vi "试剂余量后台任务.vi"   [LabVIEW 2016, in "斯坦道总氮.lvlib"]
uses:
  <vilib>/ptbypt/NI_PtbyPt.lvlib
types:
  T1 = cluster{"V1":sgl, "V2":sgl, "V3":sgl, "V4":sgl, "V5":sgl, "V6":sgl, "V7":sgl, "V8":sgl, "V9":sgl, "V10":sgl, "V11":sgl, "V12":sgl, "V9-1":sgl, "V9-2":sgl}
  T2 = cluster{"时间标识":timestamp, "设备":string, "日志信息":string, "备注":string}
  T3 = cluster{"系统时间":timestamp, "工作状态":u16, "测量模式":enum16{"待机", "连续模式", "周期模式", "定点模式", "受控模式", "手动模式"}, "告警代码":u16, "故障代码":u16, "日志代码":u16, "软件版本":u16, "F0":sgl, "F1":sgl, "F2":sgl, "F3":sgl, "T":sgl, "H":sgl, "id":u16, "flowid":u16, "量程":u16, "总磷控温温度1":sgl, "营养盐控温温度2":sgl, "ADC":sgl}
  T4 = cluster{"V1":bool, "V2":bool, "V3":bool, "V4":bool, "V5":bool, "V6":bool, "V7":bool, "V8":bool, "V9":bool, "V10":bool, "V11":bool, "V12":bool, "V9-1":bool, "V9-2":bool}
  T5 = cluster{"参数":string, "报警内容":string, "报警分析":string}
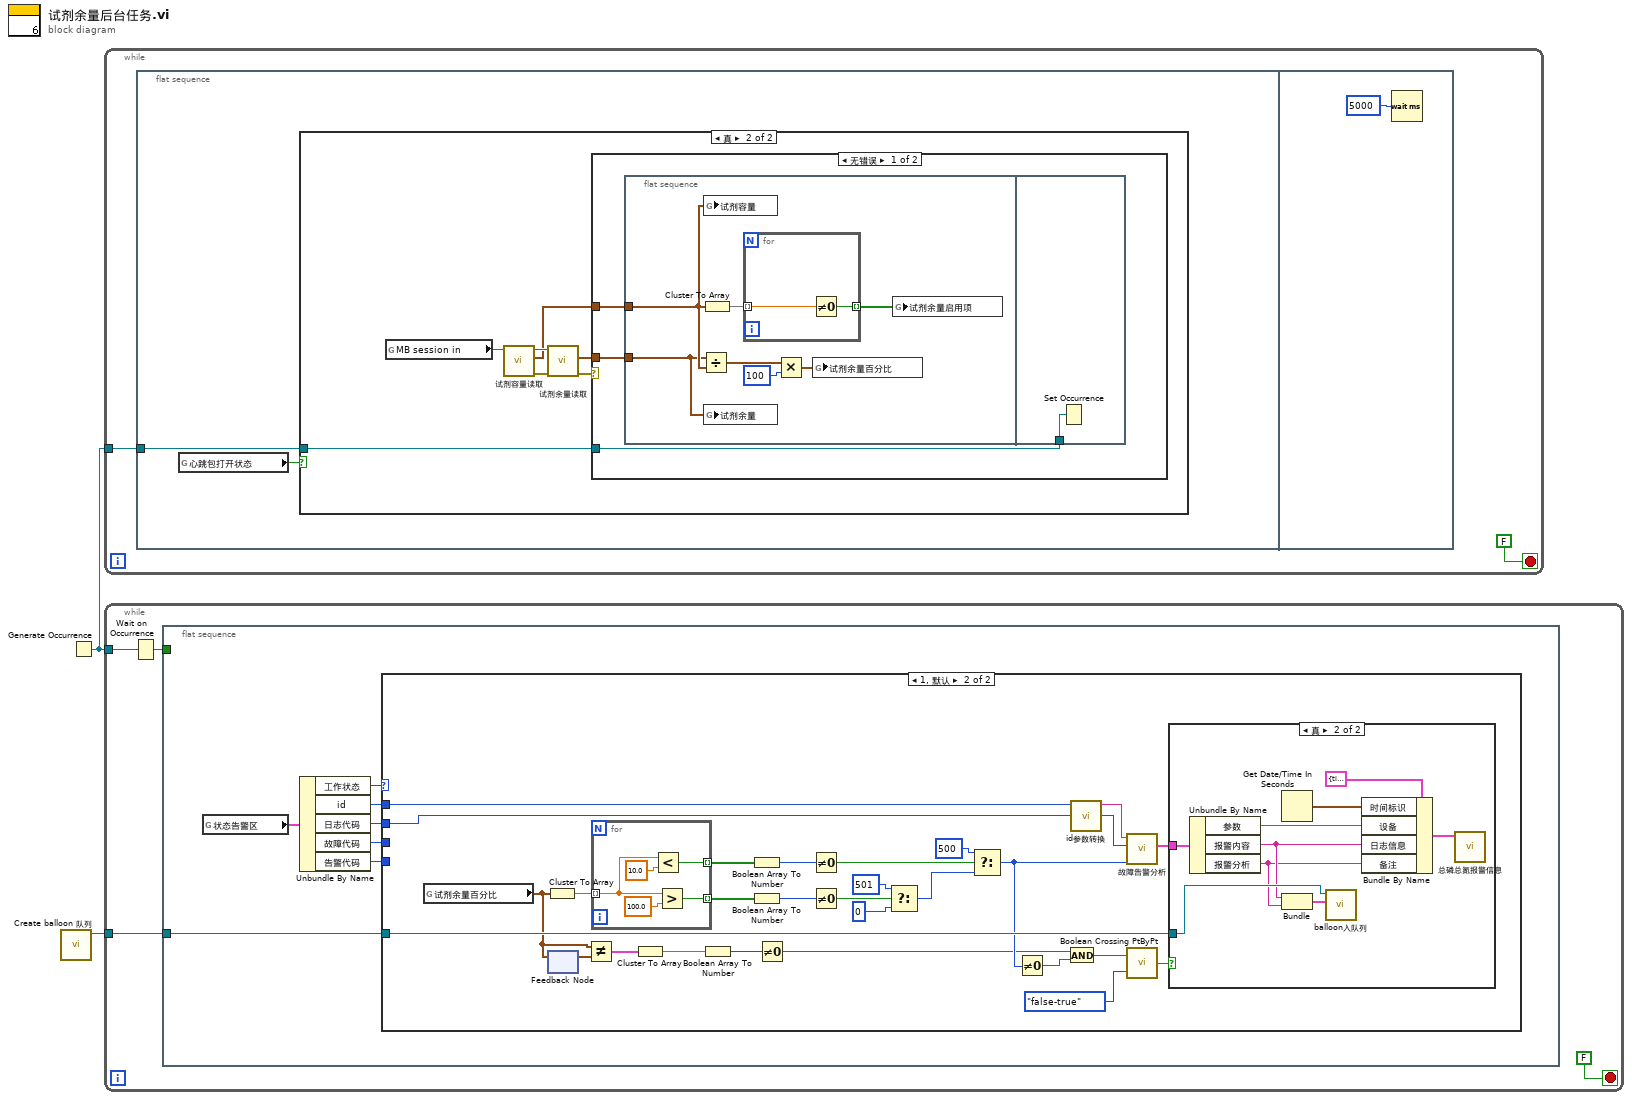
[diagram p0: block diagram]
diagram:
  n1 = call "Create balloon 队列.vi"() -> ("队列输出"=w2:refnum<queue>)  [unwired: 11 in]
  n2 = Generate Occurrence() -> (w1:refnum<k4>)
  n3 = while {
    tunnel: w1 -> [w3]
    stop <- FALSE stop-if-true
    n4 = flat-sequence {
      tunnel: w3 -> [w6]
      frame #0 {
        n5 = global read "VAR总磷总氮全局变量.vi" "心跳包打开状态"() -> (w5:bool)
        n6 = case shown="真" w5 {
          tunnel: w6 -> [_ w7]
          frame False {
          }
          frame True {
            n7 = global read "VAR总磷总氮全局变量.vi" "MB session in"() -> (w11:refnum<class "MB_Master.lvclass">)
            n8 = call "试剂容量读取.vi"("MB session in"=w11) -> ("error out"=w13:errorcluster, "试剂容量"=w10:T1, "MB session out"=w12:refnum<class "MB_Master.lvclass">)  [unwired: 8 in]
            n9 = call "试剂余量读取.vi"("Error in"=w13, "MB session in"=w12) -> ("error out"=w8:errorcluster, "试剂余量"=w9:T1)  [unwired: 7 in, 1 out]
            n10 = case shown="无错误" w8 {
              tunnel: w10 -> [w16 _]
              tunnel: w9 -> [w15 _]
              tunnel: w7 -> [w14 _]
              frame No Error {
                n11 = flat-sequence {
                  tunnel: w16 -> [w21]
                  tunnel: w15 -> [w20]
                  tunnel: w14 -> [w26]
                  frame #0 {
                    n12 = Divide(x=w20, y=w21) -> (x/y=w23:T1)
                    n13 = Cluster To Array(cluster=w21) -> (array=w18:sgl[])
                    n14 = global write "VAR总磷总氮全局变量.vi" "试剂容量"(w21) -> ()
                    n15 = global write "VAR总磷总氮全局变量.vi" "试剂余量"(w20) -> ()
                    n16 = for {
                      tunnel: w18 -> [w25] mode=indexing
                      tunnel: [w24] -> w17 mode=indexing
                      n17 = Not Equal To 0?(x=w25) -> (x != 0?=w24:bool)
                    }
                    n18 = Multiply(x=w23, y=100) -> (x*y=w19:T1)
                    n19 = global write "VAR总磷总氮全局变量.vi" "试剂余量百分比"(w19) -> ()
                    n20 = global write "VAR总磷总氮全局变量.vi" "试剂余量启用项"(w17) -> ()
                  }
                  frame #1 {
                    n21 = Set Occurrence(w26) -> ()
                  }
                }
              }
              frame Error {
              }
            }
          }
        }
      }
      frame #1 {
        n22 = Wait (ms)(milliseconds to wait=u32 5000 ("等待时间（毫秒）")) -> ()  [unwired: 1 out]
      }
    }
  }
  n23 = while {
    tunnel: w2 -> [w30]
    tunnel: w1 -> [w29]
    stop <- FALSE stop-if-true
    n24 = Wait on Occurrence(2:w29) -> (0:w28:bool)  [unwired: 2 in]
    n25 = flat-sequence {
      tunnel: w30 -> [w36]
      tunnel: w28 -> [_]
      frame #0 {
        n26 = global read "VAR总磷总氮全局变量.vi" "状态告警区"() -> (w32:T3)
        n27 = Unbundle By Name(w32) -> ("工作状态"=w33:u16, "id"=w38:u16, "日志代码"=w37:u16, "故障代码"=w35:u16, "告警代码"=w34:u16)
        n28 = case shown="1, 默认" w33 {
          tunnel: w38 -> [_ w65]
          tunnel: w37 -> [_ w64]
          tunnel: w36 -> [_ w61]
          tunnel: w35 -> [_ _]
          tunnel: w34 -> [_ _]
          frame 0 {
          }
          frame 1, Default {
            n29 = global read "VAR总磷总氮全局变量.vi" "试剂余量百分比"() -> (w46:T1)
            n30 = Cluster To Array(cluster=w46) -> (array=w56:sgl[])
            n31 = feedback-in #1(w46) -> ()
            n32 = feedback #1() -> (w47:T1)  [unwired: 1 in]
            n33 = Not Equal?(x=w46, y=w47) -> (x != y?=w45:T4)
            n34 = for {
              tunnel: w56 -> [w68] mode=indexing
              tunnel: [w69] -> w58 mode=indexing
              tunnel: [w66] -> w57 mode=indexing
              n35 = Less?(x=w68, y=sgl 10.0) -> (x < y?=w69:bool)
              n36 = Greater?(x=w68, y=sgl 100.0) -> (0:w66:bool)
            }
            n37 = Cluster To Array(cluster=w45) -> (array=w44:bool[])
            n38 = Boolean Array To Number(Boolean array=w44) -> (number=w43:u32)
            n39 = Boolean Array To Number(Boolean array=w58) -> (number=w60:u32)
            n40 = Boolean Array To Number(Boolean array=w57) -> (number=w59:u32)
            n41 = Not Equal To 0?(x=w43) -> (x != 0?=w41:bool)
            n42 = Not Equal To 0?(x=w60) -> (x != 0?=w55:bool)
            n43 = Not Equal To 0?(x=w59) -> (x != 0?=w53:bool)
            n44 = Select(t=501, s=w53, f=0) -> (s? t:f=w50:i32)
            n45 = Select(t=500, s=w55, f=w50) -> (s? t:f=w49:i32)
            n46 = Not Equal To 0?(x=w49) -> (x != 0?=w48:bool)
            n47 = And(x=w41, y=w48) -> (x .and. y?=w42:bool)
            n48 = call "id参数转换.vi"("id"=w65) -> ("table输出"=w62:string)  [unwired: 9 in, 1 out]
            n49 = call "故障告警分析.vi"("告警代码"=w49, "运行步序"=w64, "参数"=w62) -> ("报警内容"=w63:T5)  [unwired: 7 in, 1 out]
            n50 = call <vilib>:"Boolean Crossing PtByPt.vi"("direction"=enum16{"either", "false-true", "true-false"}."false-true", "input"=w42) -> ("crossing"=w40:bool)  [unwired: 1 in]
            n51 = case shown="真" w40 {
              tunnel: w63 -> [_ w79]
              tunnel: w61 -> [_ w78]
              frame False {
              }
              frame True {
                n52 = Unbundle By Name(w79) -> ("参数"=w74:string, "报警内容"=w73:string, "报警分析"=w72:string)
                n53 = Get Date/Time In Seconds() -> (seconds since 1Jan1904=w77:timestamp)
                n54 = Bundle("报警内容"=w73, "报警分析"=w72) -> (w71:cluster{"报警内容":string, "报警分析":string})  [unwired: 1 in]
                n55 = call "balloon入队列.vi"("报警内容"=w71, "队列"=w78) -> ()  [unwired: 9 in, 1 out]
                n56 = Bundle By Name(cluster=T2 {"时间标识"=timestamp(0 s since 1904-01-01), "设备"="", "日志信息"="", "备注"=""} ("data in"), "时间标识"=w77, "设备"=w74, "日志信息"=w73, "备注"=w72) -> (w76:T2)
                n57 = call "总磷总氮报警信息.vi"("data in"=w76) -> ()  [unwired: 10 in, 1 out]
              }
            }
          }
        }
      }
    }
  }
